vi "lvstyx_get_file_len.vi"(8 "error in (no error)":errorcluster, 11 "file ptr":u32) -> (0 "error out":errorcluster, 3 "length":i32)   [LabVIEW 2010, in "lib1299.lvlib"]
uses:
  lib1299.lvlib
  cstyx/win32/cstyx.dll
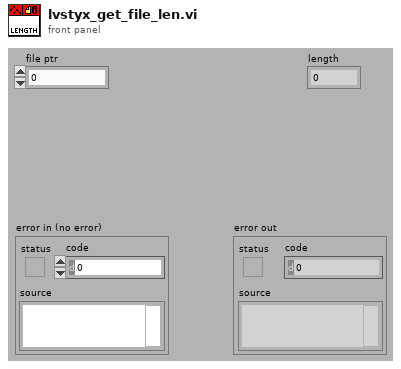
[diagram p1: front panel]
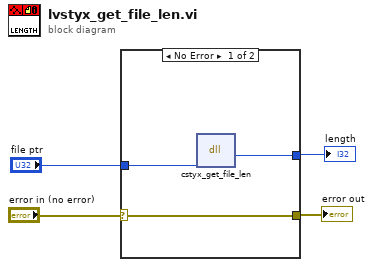
[diagram p0: block diagram]
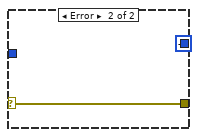
[diagram p2: hidden frame]
diagram:
  n1 = case shown="No Error" "error in (no error)" {
    selector: "error in (no error)" -> [w5 w9]
    tunnel: [w5 w9] -> w3
    tunnel: "file ptr" -> [w7 _]
    tunnel: [w6 -1 ("length")] -> w1
    frame No Error {
      n2 = dll-call lib="C:/work/ads1299evm/lib_1299/Styx/cstyx/win32/cstyx.dll" fn="cstyx_get_file_len"("file ptr"=w7) -> ("length"=w6:i32)  [unwired: 4 in, 2 out]
    }
    frame Error {
    }
  }
  "error out" <- w3
  "length" <- w1
